vi "Console_Create.vi"(8 "error in (no error)":errorcluster, 11 "reference in":refnum<class "Console.lvclass">) -> (0 "error out":errorcluster, 3 "reference out":refnum<class "Console.lvclass">)   [LabVIEW 2018, in "Console.lvclass"]
uses:
  Console.lvclass
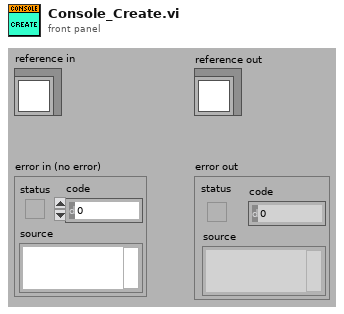
[diagram p1: front panel]
types:
  T1 = typedef "Console.lvclass/ObjectAttributes.ctl" = cluster{"data":string, "count":dbl, "ConsoleRef":refnum<vi>}
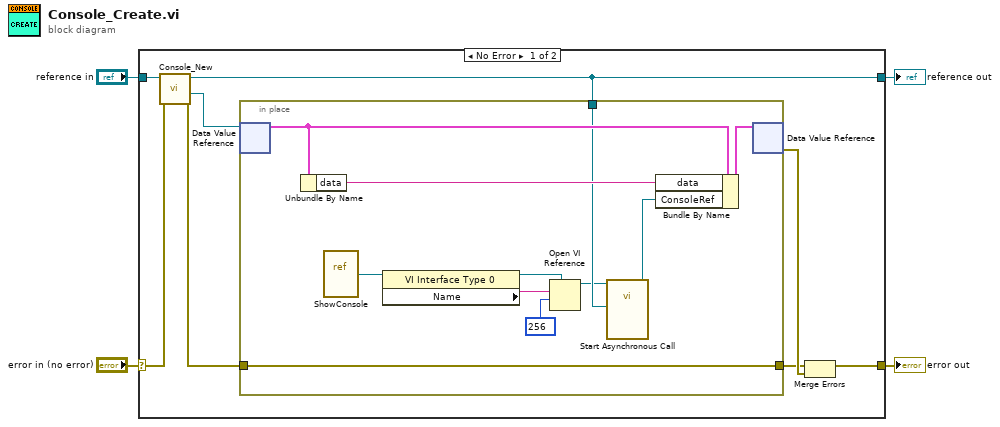
[diagram p0: block diagram]
diagram:
  n1 = case shown="No Error" "error in (no error)" {
    selector: "error in (no error)" -> [w11 w25]
    tunnel: [w6 w25] -> w3
    tunnel: "reference in" -> [w12 w24]
    tunnel: [w5 w24] -> w1
    frame No Error {
      n2 = call "Console_New.vi"("error in (no error)"=w11, "reference in"=w12) -> ("error out"=w8:errorcluster, "DVRRefOut"=w9:refnum<data-value>, "reference out"=w5:refnum<class "Console.lvclass">)  [unwired: 6 in, 1 out]
      n3 = in-place {
        in-place-border: w8 -> [w20]
        in-place-border: [w20] -> w7
        in-place-border: w5 -> [w15]
        n4 = in-place-dvr #1(w9) -> (w22:T1)  [unwired: 1 out]
        n5 = Unbundle By Name(w22) -> ("data"=w21:string)
        n6 = vi-ref "ShowConsole.vi"() -> (w19:refnum<vi>)
        n7 = property class="VI Interface Type 0"(reference=w19) -> (reference out=w17:refnum<vi>, "Name"=w18:string)  [unwired: 1 in, 1 out]
        n8 = Open VI Reference(type specifier VI Refnum (for type only)=w17, vi path=w18, options=256) -> (vi reference=w14:refnum<vi>)  [unwired: 3 in, 1 out]
        n9 = call-by-ref "Start Asynchronous Call"(reference=w14, "reference in"=w15) -> (reference out=w13:refnum<vi>)  [unwired: 10 in, 3 out]
        n10 = Bundle By Name(cluster=w22, "data"=w21, "ConsoleRef"=w13) -> (w23:T1)
        n11 = in-place-dvr #1(w23) -> (w10:errorcluster)  [unwired: 1 out]
      }
      n12 = Merge Errors(w7, w10) -> (w6:errorcluster)
    }
    frame Error {
      # "VI-TechBaseTemplate_Simple_4x4x4"
    }
  }
  "error out" <- w3
  "reference out" <- w1
